vi "Score All Combinations.vi"(10 "parsed string":u8[](array[numeric]), 11 "row map":string[](array[string])) -> (3 "arrangements":i32)   [LabVIEW 2022 SP3]
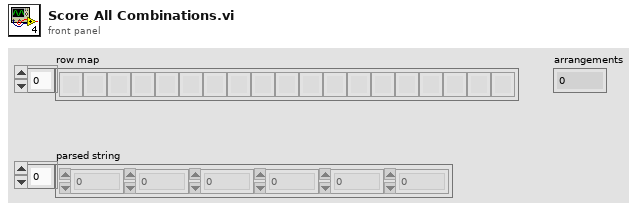
[diagram p1: front panel]
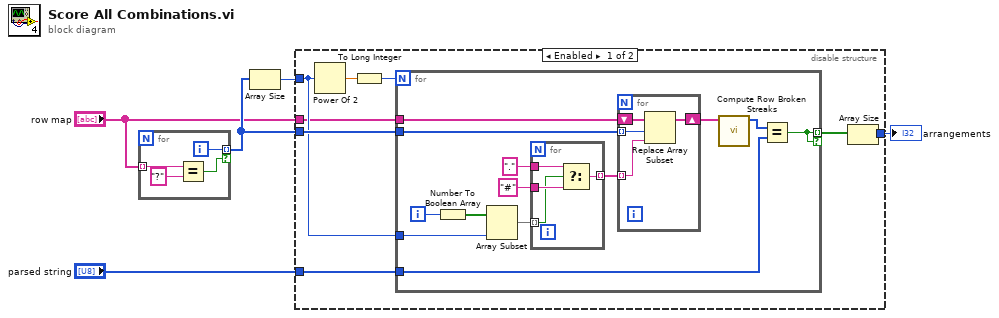
[diagram p0: block diagram]
diagram:
  n1 = for {
    tunnel: "row map" -> [w9] mode=indexing
    tunnel: [w7] -> w5 mode=indexing if=w6
    i -> [w7]
    n2 = Equal?(x=w9, y="?") -> (x = y?=w6:bool)
  }
  n3 = Array Size(array=w5) -> (size(s)=w4:i32)
  n4 = disable-structure shown="Enabled" {
    disable-tunnel: w5 -> [w15 _]
    disable-tunnel: w4 -> [w14 _]
    disable-tunnel: "parsed string" -> [w13 _]
    disable-tunnel: [w11 _] -> w2
    disable-tunnel: "row map" -> [w10 _]
    frame Enabled {
      n5 = Power Of 2(x=w14) -> (2^x=w17:dbl)
      n6 = To Long Integer(number=w17) -> (32bit integer=w16:i32)
      n7 = for {
        N: w16 -> [_]
        tunnel: w10 -> [w26]
        tunnel: w15 -> [w25]
        tunnel: w14 -> [w22]
        tunnel: w13 -> [w19]
        tunnel: [w18] -> w12 mode=indexing if=w18
        i -> [w30]
        n8 = Number To Boolean Array(number=w30) -> (Boolean array=w24:bool[])
        n9 = Array Subset(array=w24, length=w22) -> (w23:bool[])  [unwired: 1 in]
        n10 = for {
          tunnel: w23 -> [w32] mode=indexing
          tunnel: "." ("y") -> [w34]
          tunnel: "#" ("y") -> [w33]
          tunnel: [w31] -> w27 mode=indexing
          n11 = Select(t=w34, s=w32, f=w33) -> (s? t:f=w31:string)
        }
        n12 = for {
          tunnel: w27 -> [w36] mode=indexing
          tunnel: w25 -> [w37] mode=indexing
          shift-right: [w35] -> w21
          shift-left: w26 -> [w38]
          n13 = Replace Array Subset(array=w38, new element=w36, index=w37) -> (w35:string[])
        }
        n14 = call "Compute Row Broken Streaks.vi"("row map"=w21) -> ("broken streaks"=w20:u8[])  [unwired: 10 in]
        n15 = Equal?(x=w20, y=w19) -> (x = y?=w18:bool)
      }
      n16 = Array Size(array=w12) -> (size(s)=w11:i32)
    }
    frame Disabled {
    }
  }
  "arrangements" <- w2
